vi "GetForLoopCount.vi"(5 "ForLoop in":refnum<class "ForLoop.lvclass">, 6 "error in":errorcluster, 9 "VI Interpreter in":refnum<class "VI Interpreter.lvclass">) -> (0 "error out":errorcluster, 3 "VI Interpreter out":refnum<class "VI Interpreter.lvclass">, 4 "ForLoop out":refnum<class "ForLoop.lvclass">)   [LabVIEW 2014, in "Raspberry Pi Compatible Compiler for LabVIEW.lvlib" / "VI Interpreter.lvclass"]
uses:
  VI Interpreter.lvclass
  ForLoop/ForLoop.lvclass
  ForLoop/ForLoop.lvclass/ForLoop.ctl
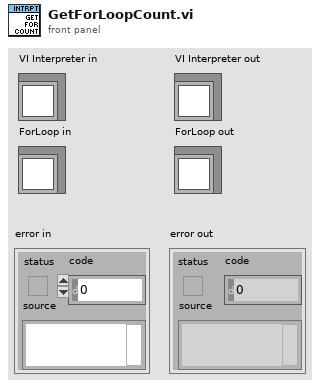
[diagram p1: front panel]
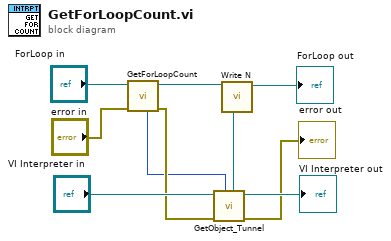
[diagram p0: block diagram]
diagram:
  n1 = call-dynamic "GetForLoopCount.vi"("error in"="error in", "ForLoop in"="ForLoop in") -> ("error out"=w4:errorcluster, "ForLoop out"=w5:refnum<class "ForLoop.lvclass">, "count UID"=w3:i32)  [unwired: 5 in]
  n2 = call "GetObject_Tunnel.vi"("UID"=w3, "error in"=w4, "VI Interpreter in"="VI Interpreter in") -> ("error out"=→"error out":errorcluster, "VI Interpreter out"=→"VI Interpreter out":refnum<class "VI Interpreter.lvclass">, "Tunnel"=w9:refnum<class "Tunnel.lvclass">)  [unwired: 3 in, 1 out]
  n3 = call "Write N.vi"("N"=w9, "ForLoop in"=w5) -> ("ForLoop out"=→"ForLoop out":refnum<class "ForLoop.lvclass">)  [unwired: 7 in]
